vi "template image save.vi"(0 "Refnum in":refnum<k21> caption="IMAQdx Session", 5 "camera":T1(plugin-control), 7 "Cross Hair Coordinates in":cluster{"X":i32, "Y":i32}, 9 "Boolean":bool, 11 "error in (no error)":errorcluster) -> (1 "Buffer Number":u32, 2 "X":dbl, 3 "Y":dbl, 4 "Refnum out":T1, 6 "Session Out":T2, 8 "Frame Rate":dbl(knob) scale=0.0..100.0, 10 "Image 2":T1(plugin-control), 13 "Particle Measurements (Pixels) 4":dbl[][](array[numeric]) format="%.2f", 14 "Particle Measurements (Pixels) 3":dbl[][](array[numeric]) format="%.2f", 15 "error out":errorcluster)   [LabVIEW 2017]
uses:
  <vilib>/vision/Image Controls.llb/IMAQ Image.ctl
  <vilib>/userdefined/High Color/IMAQdx.ctl
  <vilib>/vision/driver/NI_Vision_Acquisition_Software.lvlib
  <resource>/objmgr/imaqdx.rc
  <vilib>/vision/NI_Vision_Development_Module.lvlib
panel:
  out "Image":T1(plugin-control)
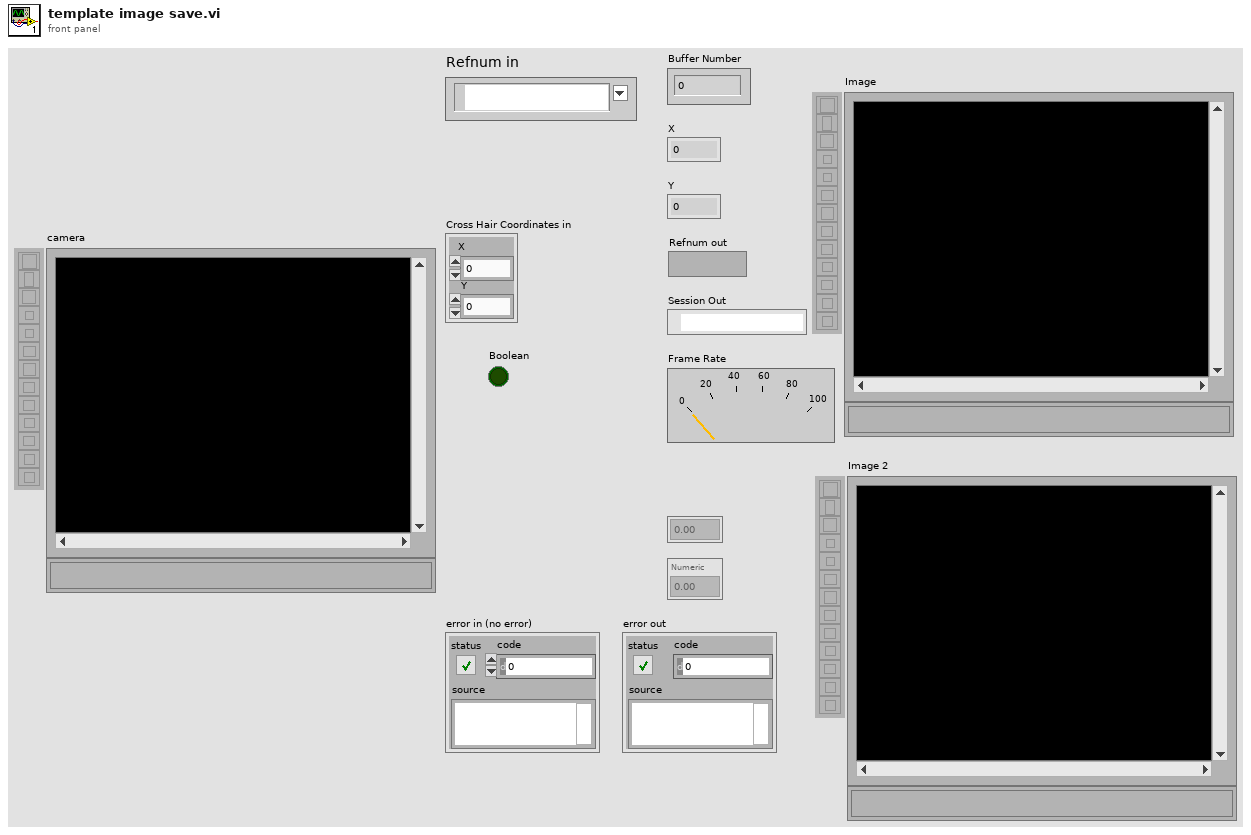
[diagram p1: front panel]
types:
  T1 = typedef "IMAQ Image.ctl" = refnum<image>
  T2 = typedef "IMAQdx.ctl" = refnum<k21>
  T3 = typedef "Image Type" = u32
  T4 = typedef "Particle Parameters" = i32
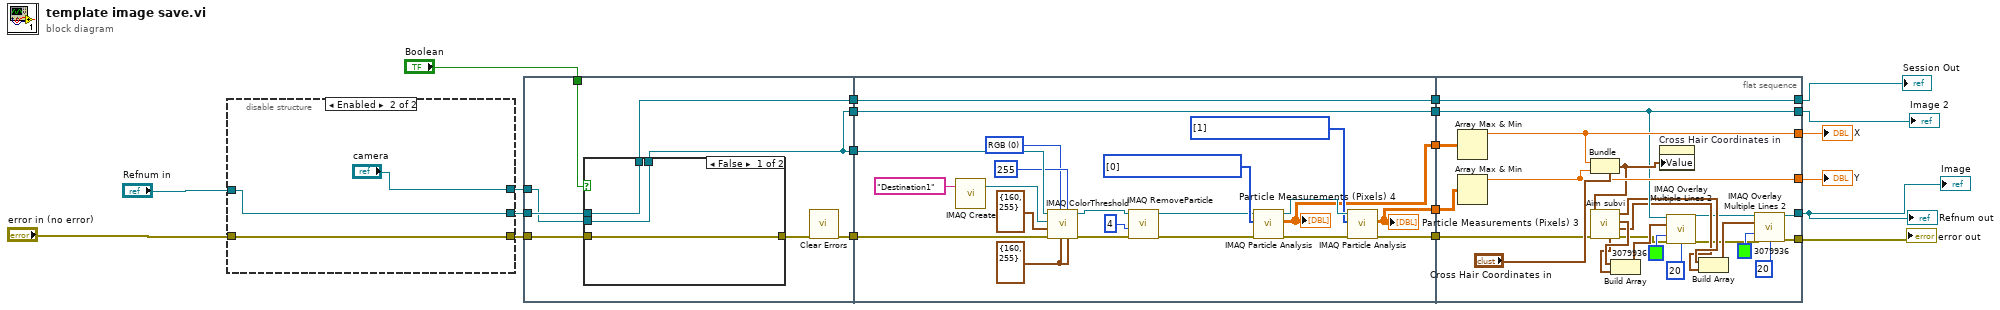
[diagram p0: block diagram]
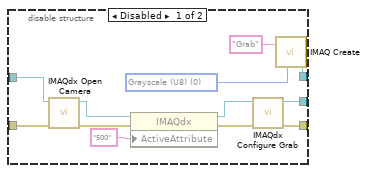
[diagram p2: hidden frame]
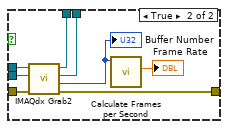
[diagram p3: hidden frame]
diagram:
  n1 = disable-structure shown="Enabled" {
    disable-tunnel: [w27 "camera"] -> w9
    disable-tunnel: [w26 w36] -> w8
    disable-tunnel: [w25 w35] -> w7
    disable-tunnel: "Refnum in" -> [w23 w36]
    disable-tunnel: "error in (no error)" -> [w22 w35]
    frame Disabled {
      w32 = T3 0 items=["Grayscale (U8)", "Grayscale (I16)", "Grayscale (SGL)", "Complex (CSG)", "RGB (U32)", "HSL (U32)", "RGB (U64)", "Grayscale (U16)"] ("Image Type")
      n2 = call <vilib>:"IMAQdx Open Camera.vi"("error in"=w22, "Session In"=w23) -> ("error out"=w29:errorcluster, "Session Out"=w28:T2)  [unwired: 1 in, 7 out]
      n3 = property class="IMAQdx"(reference=w28, error in=w29, "ActiveAttribute"="500") -> (reference out=w30:T2, error out=w33:errorcluster)
      n4 = call <vilib>:"IMAQdx Configure Grab.vi"("error in"=w33, "Session In"=w30) -> ("error out"=w25:errorcluster, "Session Out"=w26:T2)  [unwired: 8 out]
      n5 = call "IMAQ Create"("Image Name"="Grab", "Image Type"=w32) -> ("New Image"=w27:T1)  [unwired: 2 in, 2 out]
    }
    frame Enabled {
    }
  }
  n6 = flat-sequence {
    tunnel: [w44] -> w21
    tunnel: [w44] -> w20
    tunnel: [w43] -> w19
    tunnel: w9 -> [w40]
    tunnel: w8 -> [w41]
    tunnel: w7 -> [w42]
    tunnel: [w38] -> w18
    tunnel: "Boolean" -> [w37]
    tunnel: w21 -> [w64]
    tunnel: [w72] -> w17
    tunnel: [w67] -> w16
    tunnel: [w68] -> w15
    tunnel: [w71] -> w14
    tunnel: w20 -> [w71]
    tunnel: [w66] -> w13
    tunnel: w19 -> [w66]
    tunnel: w18 -> [w63]
    tunnel: w17 -> [w100]
    tunnel: w16 -> [w99]
    tunnel: w15 -> [w98]
    tunnel: w14 -> [w93]
    tunnel: w13 -> [w97]
    tunnel: [w97] -> w10
    tunnel: [w93] -> w1
    tunnel: [w81] -> w3
    tunnel: [w96] -> w11
    tunnel: [w95] -> w12
    tunnel: [w78] -> w4
    frame #0 {
      n7 = case shown="False" w37 {
        tunnel: [w46 w55] -> w44
        tunnel: [w45 w54] -> w43
        tunnel: w42 -> [w47 w51]
        tunnel: w41 -> [w45 w50]
        tunnel: w40 -> [w46 w49]
        tunnel: [w47 w48] -> w39
        frame False {
        }
        frame True {
          n8 = call <vilib>:"IMAQdx Grab2.vi"("error in"=w51, "Image In"=w49, "Session In"=w50) -> ("error out"=w48:errorcluster, "Buffer Number Out"=w52:u32, "Image Out"=w55:T1, "Session Out"=w54:T2)  [unwired: 5 in]
          "Buffer Number" <- w52
          n9 = call <vilib>:"Calculate Frames per Second.vi"("Buffer Number"=w52) -> ("Processed Frames/s"=→"Frame Rate":dbl)  [unwired: 8 in, 2 out]
        }
      }
      n10 = call <vilib>:"Clear Errors.vi"("error in (no error)"=w39) -> ("error out"=w38:errorcluster)  [unwired: 5 in, 1 out]
    }
    frame #1 {
      w56 = u16 0 items=["RGB", "HSL", "HSV", "HSI"] ("Color Mode")
      w74 = T4[] [1] items=["Center of Mass X", "Center of Mass Y", "First Pixel X", "First Pixel Y", "Bounding Rect Left", "Bounding Rect Top", "Bounding Rect Right", "Bounding Rect Bottom", "Max Feret Diameter Start X", "Max Feret Diameter Start Y", "Max Feret Diameter End X", "Max Feret Diameter End Y", "Max Horiz. Segment Length Left", "Max Horiz. Segment Length Right", "Max Horiz. Segment Length Row", "-", "Bounding Rect Width", "Bounding Rect Height", "Bounding Rect Diagonal", "Perimeter", "Convex Hull Perimeter", "Holes' Perimeter", "Max Feret Diameter", "Equivalent Ellipse Major Axis", "Equivalent Ellipse Minor Axis", "Equivalent Ellipse Minor Axis (Feret)", "Equivalent Rect Long Side", "Equivalent Rect Short Side", "Equivalent Rect Diagonal", "Equivalent Rect Short Side (Feret)", "Average Horiz. Segment Length", "Average Vert. Segment Length", "Hydraulic Radius", "Waddel Disk Diameter", "-", "Area", "Holes' Area", "Particle & Holes' Area", "Convex Hull Area", "Image Area", "-", "Number of Holes", "Number of Horiz. Segments", "Number of Vert. Segments", "-", "Orientation", "Max Feret Diameter Orientation", "-", "% Area/Image Area", "% Area/(Particle & Holes' Area)", "Ratio of Equivalent Ellipse Axes", "Ratio of Equivalent Rect Sides", "-", "Elongation Factor", "Compactness Factor", "Heywood Circularity Factor", "Type Factor", "-", "Sum X", "Sum Y", "Sum XX", "Sum XY", "Sum YY", "Sum XXX", "Sum XXY", "Sum XYY", "Sum YYY", "-", "Moment of Inertia XX", "Moment of Inertia XY", "Moment of Inertia YY", "Moment of Inertia XXX", "Moment of Inertia XXY", "Moment of Inertia XYY", "Moment of Inertia YYY", "Norm. Moment of Inertia XX", "Norm. Moment of Inertia XY", "Norm. Moment of Inertia YY", "Norm. Moment of Inertia XXX", "Norm. Moment of Inertia XXY", "Norm. Moment of Inertia XYY", "Norm. Moment of Inertia YYY", "Hu Moment 1", "Hu Moment 2", "Hu Moment 3", "Hu Moment 4", "Hu Moment 5", "Hu Moment 6", "Hu Moment 7"] ("Pixel Measurements")
      w59 = cluster{"Lower value":i32, "Upper value":i32} {"Lower value"=160, "Upper value"=255} ("Red or Hue Range")
      w77 = T4[] [0] items=["Center of Mass X", "Center of Mass Y", "First Pixel X", "First Pixel Y", "Bounding Rect Left", "Bounding Rect Top", "Bounding Rect Right", "Bounding Rect Bottom", "Max Feret Diameter Start X", "Max Feret Diameter Start Y", "Max Feret Diameter End X", "Max Feret Diameter End Y", "Max Horiz. Segment Length Left", "Max Horiz. Segment Length Right", "Max Horiz. Segment Length Row", "-", "Bounding Rect Width", "Bounding Rect Height", "Bounding Rect Diagonal", "Perimeter", "Convex Hull Perimeter", "Holes' Perimeter", "Max Feret Diameter", "Equivalent Ellipse Major Axis", "Equivalent Ellipse Minor Axis", "Equivalent Ellipse Minor Axis (Feret)", "Equivalent Rect Long Side", "Equivalent Rect Short Side", "Equivalent Rect Diagonal", "Equivalent Rect Short Side (Feret)", "Average Horiz. Segment Length", "Average Vert. Segment Length", "Hydraulic Radius", "Waddel Disk Diameter", "-", "Area", "Holes' Area", "Particle & Holes' Area", "Convex Hull Area", "Image Area", "-", "Number of Holes", "Number of Horiz. Segments", "Number of Vert. Segments", "-", "Orientation", "Max Feret Diameter Orientation", "-", "% Area/Image Area", "% Area/(Particle & Holes' Area)", "Ratio of Equivalent Ellipse Axes", "Ratio of Equivalent Rect Sides", "-", "Elongation Factor", "Compactness Factor", "Heywood Circularity Factor", "Type Factor", "-", "Sum X", "Sum Y", "Sum XX", "Sum XY", "Sum YY", "Sum XXX", "Sum XXY", "Sum XYY", "Sum YYY", "-", "Moment of Inertia XX", "Moment of Inertia XY", "Moment of Inertia YY", "Moment of Inertia XXX", "Moment of Inertia XXY", "Moment of Inertia XYY", "Moment of Inertia YYY", "Norm. Moment of Inertia XX", "Norm. Moment of Inertia XY", "Norm. Moment of Inertia YY", "Norm. Moment of Inertia XXX", "Norm. Moment of Inertia XXY", "Norm. Moment of Inertia XYY", "Norm. Moment of Inertia YYY", "Hu Moment 1", "Hu Moment 2", "Hu Moment 3", "Hu Moment 4", "Hu Moment 5", "Hu Moment 6", "Hu Moment 7"] ("Pixel Measurements")
      n11 = call "IMAQ Create"("Image Name"="Destination1") -> ("New Image"=w61:T1)  [unwired: 3 in, 2 out]
      n12 = call "IMAQ ColorThreshold"("Blue or Luma or Val or Inten Range"=w59, "Replace Value"=255, "Green or Sat Range"=w59, "Color Mode"=w56, "error in (no error)"=w63, "Red or Hue Range"=cluster{"Lower value":i32, "Upper value":i32} {"Lower value"=160, "Upper value"=255}, "Image Dst"=w61, "Image Src"=w64) -> ("error out"=w62:errorcluster, "Image Dst Out"=w58:T1)  [unwired: 2 in]
      n13 = call "IMAQ RemoveParticle"("error in (no error)"=w62, "Number of Erosion"=4, "Image Src"=w58) -> ("error out"=w65:errorcluster, "Image Dst Out"=w70:T1)  [unwired: 4 in, 3 out]
      n14 = call "IMAQ Particle Analysis"("error in (no error)"=w65, "Pixel Measurements"=w77, "Image"=w70) -> ("error out"=w73:errorcluster, "Particle Measurements (Pixels)"=w67:dbl[][], "Image Out (duplicate)"=w75:T1)  [unwired: 3 in, 3 out]
      "Particle Measurements (Pixels) 4" <- w67
      n15 = call "IMAQ Particle Analysis"("error in (no error)"=w73, "Pixel Measurements"=w74, "Image"=w75) -> ("error out"=w72:errorcluster, "Particle Measurements (Pixels)"=w68:dbl[][])  [unwired: 3 in, 4 out]
      "Particle Measurements (Pixels) 3" <- w68
    }
    frame #2 {
      n16 = Array Max & Min(array=w99) -> (max value=w95:dbl)  [unwired: 3 out]
      n17 = Array Max & Min(array=w98) -> (max value=w96:dbl)  [unwired: 3 out]
      n18 = Bundle(cluster="Cross Hair Coordinates in", "X"=w95, "Y"=w96) -> (w94:cluster{"X":i32, "Y":i32})
      n19 = call "Aim subvi.vi"("Coordinates"=w94, "error in (no error)"=w100) -> ("Cluster 3"=w91:cluster{"X":i32, "Y":i32}, "Cluster 2"=w85:cluster{"X":i32, "Y":i32}, "Cluster 4"=w92:cluster{"X":i32, "Y":i32}, "Cluster"=w84:cluster{"X":i32, "Y":i32}, "error out"=w80:errorcluster)  [unwired: 4 in]
      n20 = Build Array(w92, w91) -> (w90:cluster{"X":i32, "Y":i32}[])
      n21 = property on="Cross Hair Coordinates in" class="Clust (strict)"("Value"=w94) -> ()  [unwired: 2 in, 2 out]
      n22 = call "IMAQ Overlay Multiple Lines 2"("Image"=w93, "Line End Points"=w90, "Color"=u32 3079936, "error in (no error)"=w80, "Width"=u32 20) -> ("Image Out"=w82:T1, "error out"=w79:errorcluster)  [unwired: 9 in]
      n23 = Build Array(w85, w84) -> (w83:cluster{"X":i32, "Y":i32}[])
      n24 = call "IMAQ Overlay Multiple Lines 2"("Image"=w82, "Line End Points"=w83, "Color"=u32 3079936, "error in (no error)"=w79, "Width"=u32 20) -> ("Image Out"=w81:T1, "error out"=w78:errorcluster)  [unwired: 9 in]
    }
  }
  "X" <- w12
  "Y" <- w11
  "Refnum out" <- w3
  "error out" <- w4
  "Session Out" <- w10
  "Image" <- w3
  "Image 2" <- w1
